vi "initialization.vi"(8 "错误输入（无错误）":errorcluster, 11 "Setting":T3 {"X Pos." scale=-5.0..5.0; "Y Pos." scale=-5.0..5.0}) -> (0 "error out":errorcluster caption="错误输出", 2 "Image":T1, 3 "Status":T2 {"Setting"."X Pos." scale=-5.0..5.0; "Setting"."Y Pos." scale=-5.0..5.0})   [LabVIEW 2013]
uses:
  Setting.ctl
  init-status.ctl
  event-package.ctl
  Event1.ctl
  data-package.ctl
  Event.ctl
  imaging/Image.ctl
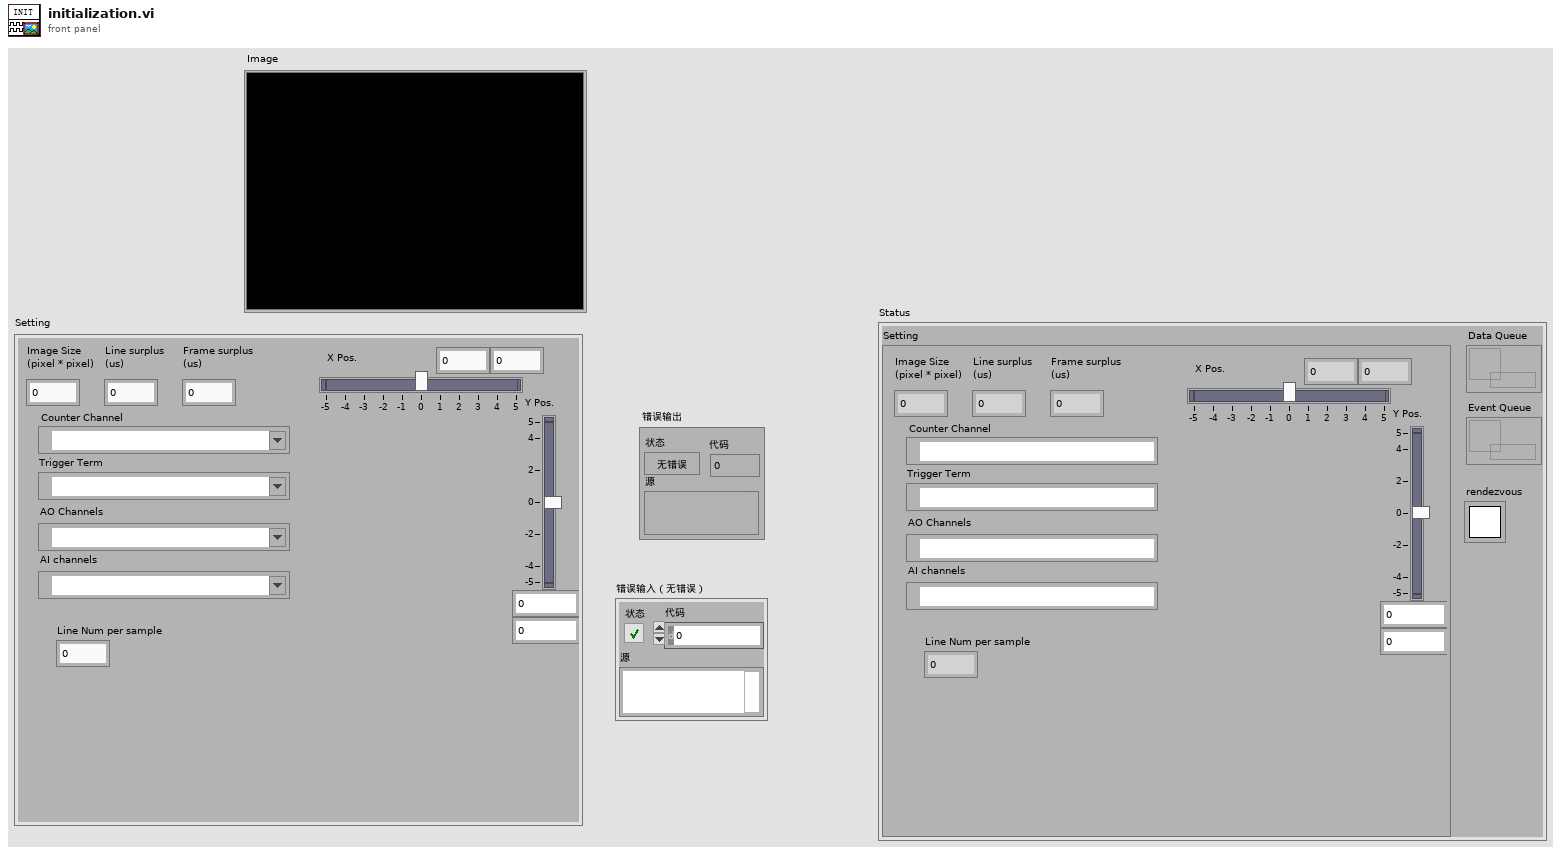
[diagram p1: front panel]
types:
  T1 = typedef "Image.ctl" = dbl[][]
  T2 = typedef "init-status.ctl" = cluster{"Setting":T3, "Event Queue":refnum<queue>, "Data Queue":refnum<queue>, "rendezvous":T4}
  T3 = typedef "Setting.ctl" = cluster{"Image Size\n(pixel * pixel)":i32, "Counter Channel":tag, "Trigger Term":tag, "AO Channels":tag, "Y Pos.":cluster{dbl, dbl}, "X Pos.":cluster{dbl, dbl}, "Line surplus\n(us)":i32, "Frame surplus\n(us)":i32, "AI channels":tag, "Line Num per sample":i32}
  T4 = typedef "Rendezvous RefNum" = refnum<k1>
  T5 = typedef "event-package.ctl" = cluster{"Event":T6, "Data":string}
  T6 = typedef "Event1.ctl" = enum16{"null", "stop AI", "stop AO", "stop Imaging", "stop Counter", "save", "restart"}
  T7 = typedef "data-package.ctl" = cluster{"Event":T8, "Data":dbl[], "line #":i32}
  T8 = typedef "Event.ctl" = u16
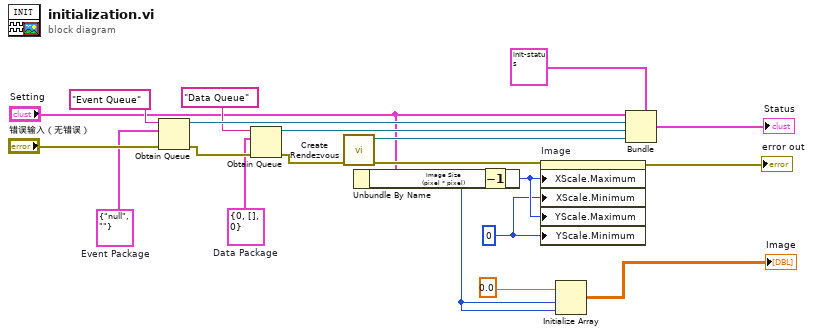
[diagram p0: block diagram]
diagram:
  w3 = 0
  w9 = T5 {"Event"=enum."null", "Data"=""}  # Event Package
  w10 = T7 {"Event"=0, "Data"=[], "line #"=0}  # Data Package
  n1 = Obtain Queue(name (unnamed)="Event Queue" ("名称（未命名）"), element data type=w9, error in (no error)="错误输入（无错误）") -> (queue out=w20:refnum<queue>, error out=w17:errorcluster)  [unwired: 2 in, 1 out]
  n2 = Obtain Queue(name (unnamed)="Data Queue" ("名称（未命名）"), element data type=w10, error in (no error)=w17) -> (queue out=w19:refnum<queue>, error out=w16:errorcluster)  [unwired: 2 in, 1 out]
  n3 = call <vilib>:"Create Rendezvous.vi"("error in (no error)"=w16) -> ("error out"=w14:errorcluster, "rendezvous"=w18:T4)  [unwired: 4 in, 1 out]
  n4 = Unbundle By Name("Setting") -> ("Image Size\n(pixel * pixel)"=w4:i32)
  n5 = Decrement(x=w4) -> (x-1=w5:i32)
  n6 = property on="Image" class="IntGraph (严格)"(error in=w14, "XScale.Maximum"=w5, "XScale.Minimum"=w3, "YScale.Maximum"=w5, "YScale.Minimum"=w3) -> (error out=→"error out":errorcluster)  [unwired: 1 in, 1 out]
  n7 = Initialize Array(0.0, w4, w4) -> (→"Image":dbl[][])
  n8 = Bundle(cluster=T2 {"Setting"={"Image Size\n(pixel * pixel)"=0, "Counter Channel"="", "Trigger Term"="", "AO Channels"="", "Y Pos."={0.0, 0.0}, "X Pos."={0.0, 0.0}, "Line surplus\n(us)"=0, "Frame surplus\n(us)"=0, "AI channels"="", "Line Num per sample"=0}, "Event Queue"=refnum, "Data Queue"=refnum, "rendezvous"=refnum} ("Status"), "Setting"="Setting", "Event Queue"=w20, "Data Queue"=w19, "rendezvous"=w18) -> (→"Status":T2)
